vi "Write to File.vi"(8 "error in":errorcluster, 10 "text":string, 11 "refnum":refnum<file>) -> (0 "error out":errorcluster, 3 "refnum out":refnum<file>)   [LabVIEW 2017]
doc: "Writes the text you specify to the file that the Create File VI created. \n\nUse this VI as the VI under test for Write to File.lvtest."
panel:
  # "Overview: Use this VI as the VI under test for Write to File.lvtest.\nRequirements: LabVIEW Full Development System, Unit Test Framework Toolkit\nInstructions: \n1.  Execute the Write to File.lvtest test file for this VI. In the Project Explorer window, right-click Write to File.lvtest, and select Run from the shortcut menu.\n2.  In the Project Explorer window, double-click Write to File.lvtest to display the Test Properties dialog box.\n3.  Select Setup/Teardown from the Category list to display the Setup/Teardown page. You can understand how LabVIEW passes values among the setup VI, the VI under test, and the teardown VI."
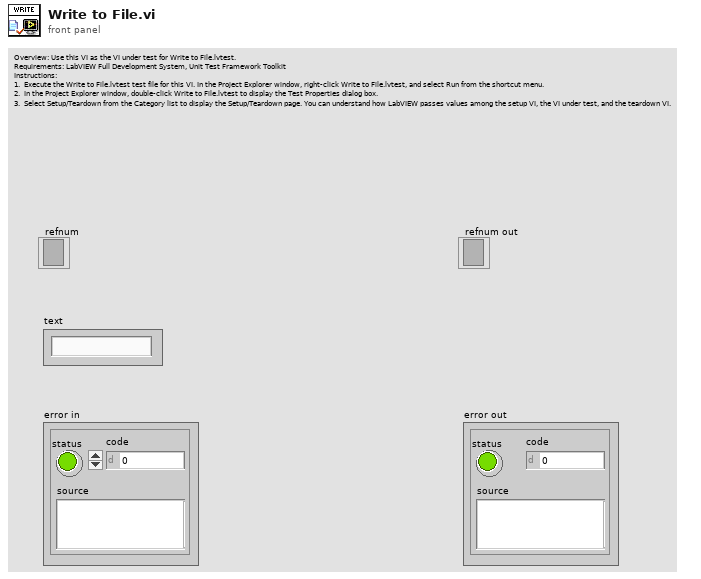
[diagram p1: front panel]
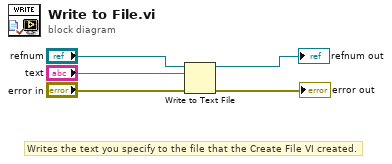
[diagram p0: block diagram]
diagram:
  # "Writes the text you specify to the file that the Create File VI created."
  n1 = Write to Text File(file (use dialog)="refnum", text="text", error in="error in") -> (refnum out=→"refnum out":refnum<file>, error out=→"error out":errorcluster)  [unwired: 2 out]
